vi "Dig a Grave - Simple.vi"() -> ()   [LabVIEW 2017]
doc: "A demonstration of digging a grave around a simple example of legacy code to be refactored. This includes step-by-step instructions for creating a grave in one of two methods: shortcut menu plugin or Quick Drop shortcut plugin. A \"grave\" is a Diagram Disable Structure with a \"Corpse\" disabled frame for the legacy code and a \"Spirit\" enabled frame with a copy of the legacy code to safely refactor."
panel:
  out "Any?":bool
  in  "Input":bool[](array[boolean])=[FALSE, FALSE, FALSE, FALSE, FALSE, FALSE, TRUE, FALSE, FALSE, FALSE]
  # "Overview: Demonstrates digging a grave for code that is to be refactored\nInstructions:\n1. Run the VI\n2. Observe the value of the Any? indicator\n3. Uncheck the TRUE element in the Input array\n4. Run the VI\n5. Observe the value of the Any? indicator\n6. Switch to the block diagram and follow the instructions there to refactor the code"
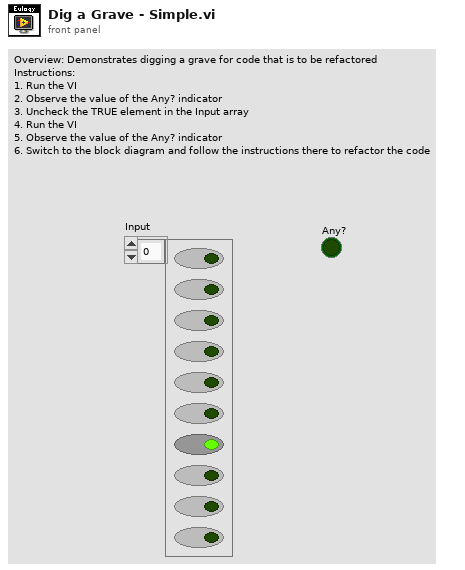
[diagram p1: front panel]
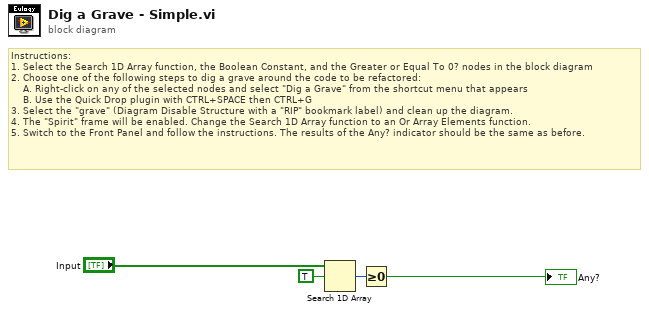
[diagram p0: block diagram]
diagram:
  # "Instructions:\n1. Select the Search 1D Array function, the Boolean Constant, and the Greater or Equal To 0? nodes in the block diagram\n2. Choose one of the following steps to dig a grave around the code to be refactored:\n    A. Right-click on any of the selected nodes and select \"Dig a Grave\" from the shortcut menu that appears\n    B. Use the Quick Drop plugin with CTRL+SPACE then CTRL+G\n3. Select the \"grave\" (Diagram Disable Structure with a \"RIP\" bookmark label) and clean up the diagram.\n4. The \"Spirit\" frame will be enabled. Change the Search 1D Array function to an Or Array Elements function. \n5. Switch to the Front Panel and follow the instructions. The results of the Any? indicator should be the same as before."
  n1 = Search 1D Array(1D array="Input", element=TRUE) -> (index of element=w1:i32)  [unwired: 1 in]
  n2 = Greater Or Equal To 0?(x=w1) -> (x >= 0?=→"Any?":bool)
